vi "StartTriggers.vi"(8 "Error In":errorcluster, 10 "Trigger Configuration":T1={"Input"={"Type"=enum."None", "Timeout (ms)"=0, "Delay (ms)"=0, "Digital IO Line (1-14)"=0, "Digital IO Mode"=enum."Falling"}, "Output"={"Type"=enum."None", "Delay (ms)"=0, "Digital IO Line (1-14)"=1, "Digital IO Mode"=enum."Falling", "Digital IO Pulse Width (sec)"=0.0}} {"Output"."Digital IO Line (1-14)" min=1 max=14 step=1}, 11 "Keithley 2602 In":refnum<visa-resource-name>) -> (0 "Error Out":errorcluster, 3 "Keithley 2602 Out":refnum<visa-resource-name>)   [LabVIEW 2012]
uses:
  TriggerConfiguration.ctl
  TriggerInputConfiguration.ctl
  TriggerInputType.ctl
  driver/Public/Controls/TriggerMode.ctl
  TriggerOutputConfiguration.ctl
  TriggerOutputType.ctl
  driver/Keithley-2602.lvlib
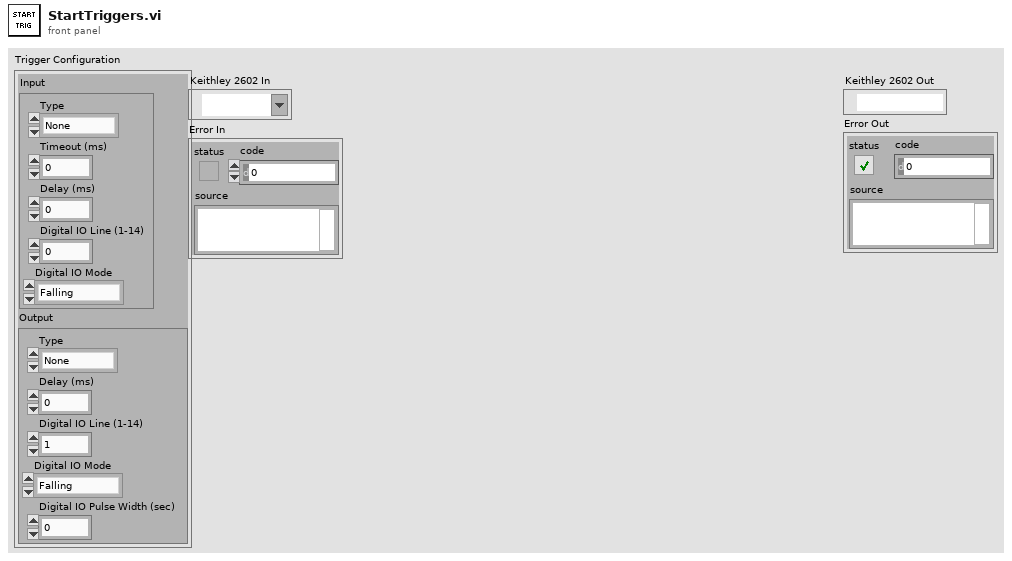
[diagram p1: front panel]
types:
  T1 = typedef "TriggerConfiguration.ctl" = cluster{"Input":T2, "Output":T5}
  T2 = typedef "TriggerInputConfiguration.ctl" = cluster{"Type":T3, "Timeout (ms)":u32, "Delay (ms)":u32, "Digital IO Line (1-14)":u8, "Digital IO Mode":T4}
  T3 = typedef "TriggerInputType.ctl" = enum16{"None", "Digital IO", "Bus"}
  T4 = typedef "Keithley-2602.lvlib/TriggerMode.ctl" = enum16{"Falling", "Rising", "Either", "Synchronous"}
  T5 = typedef "TriggerOutputConfiguration.ctl" = cluster{"Type":T6, "Delay (ms)":u32, "Digital IO Line (1-14)":u8, "Digital IO Mode":T4, "Digital IO Pulse Width (sec)":dbl}
  T6 = typedef "TriggerOutputType.ctl" = enum16{"None", "Digital IO", "Bus"}
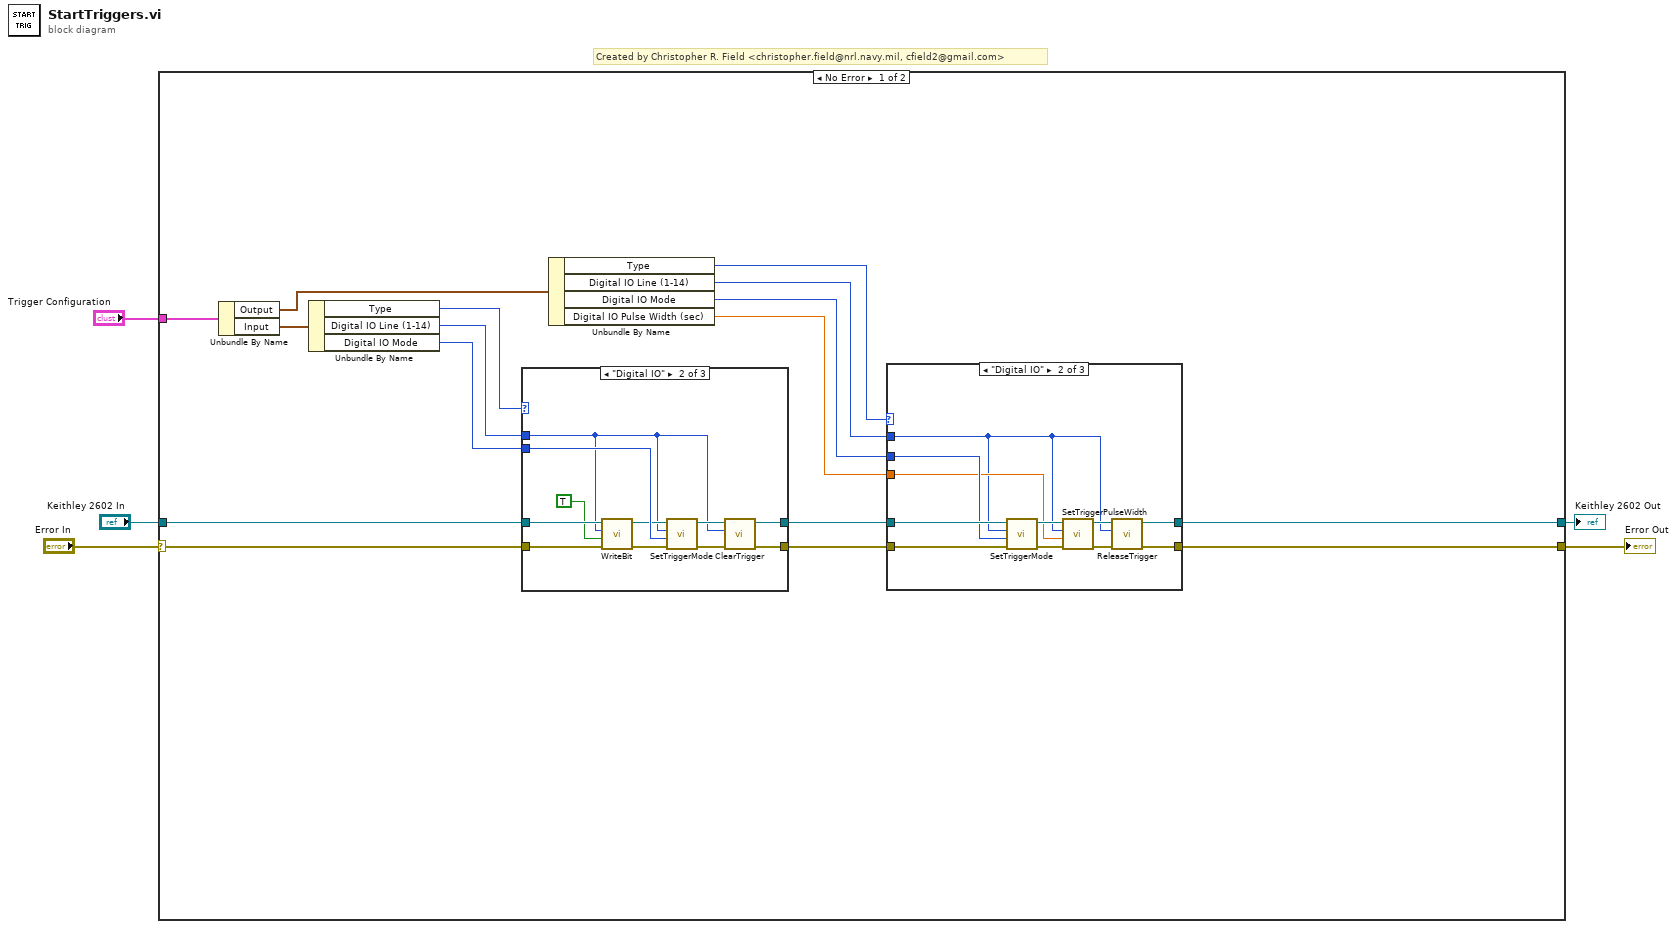
[diagram p0: block diagram]
diagram:
  # "Created by Christopher R. Field <christopher.field@nrl.navy.mil, cfield2@gmail.com>"
  n1 = case shown="No Error" "Error In" {
    selector: "Error In" -> [w6 w52]
    tunnel: "Trigger Configuration" -> [w21 _]
    tunnel: "Keithley 2602 In" -> [w7 w53]
    tunnel: [w12 w53] -> w2
    tunnel: [w11 w52] -> w1
    frame No Error {
      n2 = Unbundle By Name(w21) -> ("Output"=w17:T5, "Input"=w20:T2)
      n3 = Unbundle By Name(w20) -> ("Type"=w19:T3, "Digital IO Line (1-14)"=w18:u8, "Digital IO Mode"=w10:T4)
      n4 = case shown="\"Digital IO\"" w19 {
        tunnel: w18 -> [_ w40 _]
        tunnel: w7 -> [w38 w44 w51]
        tunnel: w6 -> [w37 w41 w50]
        tunnel: [w38 w48 w51] -> w15
        tunnel: [w37 w47 w50] -> w14
        tunnel: w10 -> [_ w49 _]
        frame "None", Default {
        }
        frame "Digital IO" {
          n5 = call "WriteBit.vi"("Error In"=w41, "State"=TRUE, "Line (1-14)"=w40, "Keithley 2602 In"=w44) -> ("Error Out"=w42:errorcluster, "Keithley 2602 Out"=w43:refnum<visa-resource-name>)  [unwired: 6 in]
          n6 = call "SetTriggerMode.vi"("Error In"=w42, "Trigger Mode"=w49, "Line (1-14)"=w40, "Keithley 2602 In"=w43) -> ("Error Out"=w45:errorcluster, "Keithley 2602 Out"=w46:refnum<visa-resource-name>)  [unwired: 6 in]
          n7 = call "ClearTrigger.vi"("Error In"=w45, "Line (1-14)"=w40, "Keithley 2602 In"=w46) -> ("Error Out"=w47:errorcluster, "Keithley 2602 Out"=w48:refnum<visa-resource-name>)  [unwired: 7 in]
        }
        frame "Bus" {
        }
      }
      n8 = Unbundle By Name(w17) -> ("Type"=w16:T6, "Digital IO Line (1-14)"=w13:u8, "Digital IO Mode"=w9:T4, "Digital IO Pulse Width (sec)"=w8:dbl)
      n9 = case shown="\"Digital IO\"" w16 {
        tunnel: w15 -> [w23 w34 w36]
        tunnel: w14 -> [w22 w33 w35]
        tunnel: w13 -> [_ w27 _]
        tunnel: [w23 w24 w36] -> w12
        tunnel: [w22 w25 w35] -> w11
        tunnel: w9 -> [_ w30 _]
        tunnel: w8 -> [_ w29 _]
        frame "None", Default {
        }
        frame "Digital IO" {
          n10 = call "SetTriggerMode.vi"("Error In"=w33, "Trigger Mode"=w30, "Line (1-14)"=w27, "Keithley 2602 In"=w34) -> ("Error Out"=w32:errorcluster, "Keithley 2602 Out"=w31:refnum<visa-resource-name>)  [unwired: 6 in]
          n11 = call "SetTriggerPulseWidth.vi"("Error In"=w32, "Pulse Width (sec)"=w29, "Line (1-14)"=w27, "Keithley 2602 In"=w31) -> ("Error Out"=w26:errorcluster, "Keithley 2602 Out"=w28:refnum<visa-resource-name>)  [unwired: 6 in]
          n12 = call "ReleaseTrigger.vi"("Error In"=w26, "Line (1-14)"=w27, "Keithley 2602 In"=w28) -> ("Error Out"=w25:errorcluster, "Keithley 2602 Out"=w24:refnum<visa-resource-name>)  [unwired: 7 in]
        }
        frame "Bus" {
        }
      }
    }
    frame Error {
    }
  }
  "Keithley 2602 Out" <- w2
  "Error Out" <- w1
